vi "Kinect_to_pixels.vi"(0 "previous_X_pixels":dbl, 1 "current_X_kinect":dbl, 2 "previous_X_kinect":dbl, 3 "previous_Y_pixels":dbl, 4 "current_Y_kinect":dbl, 5 "previous_Y_kinect":dbl, 7 "X_Y_speed":dbl, 9 "min_diff":dbl) -> (14 "X_pixels":dbl, 15 "Y_pixels":dbl, 17 "Xmax":dbl=2.5, 18 "Ymax":dbl)   [LabVIEW 2011]
panel:
  out "X_resolution":i16
  out "Y_resolution":i16
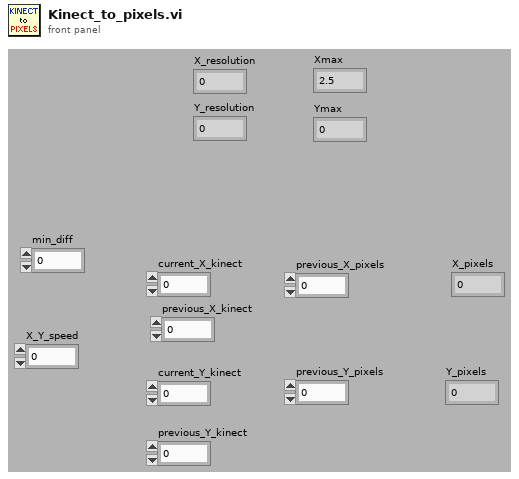
[diagram p1: front panel]
types:
  T1 = typedef "LVAllMonitorsDisplayTypeDef.ctl" = cluster{"Bounds":cluster{"Left":i16, "Top":i16, "Right":i16, "Bottom":i16}, "Depth":i16}[]
  T2 = cluster{"Bounds":cluster{"Left":i16, "Top":i16, "Right":i16, "Bottom":i16}, "Depth":i16}
  T3 = cluster{"Left":i16, "Top":i16, "Right":i16, "Bottom":i16}
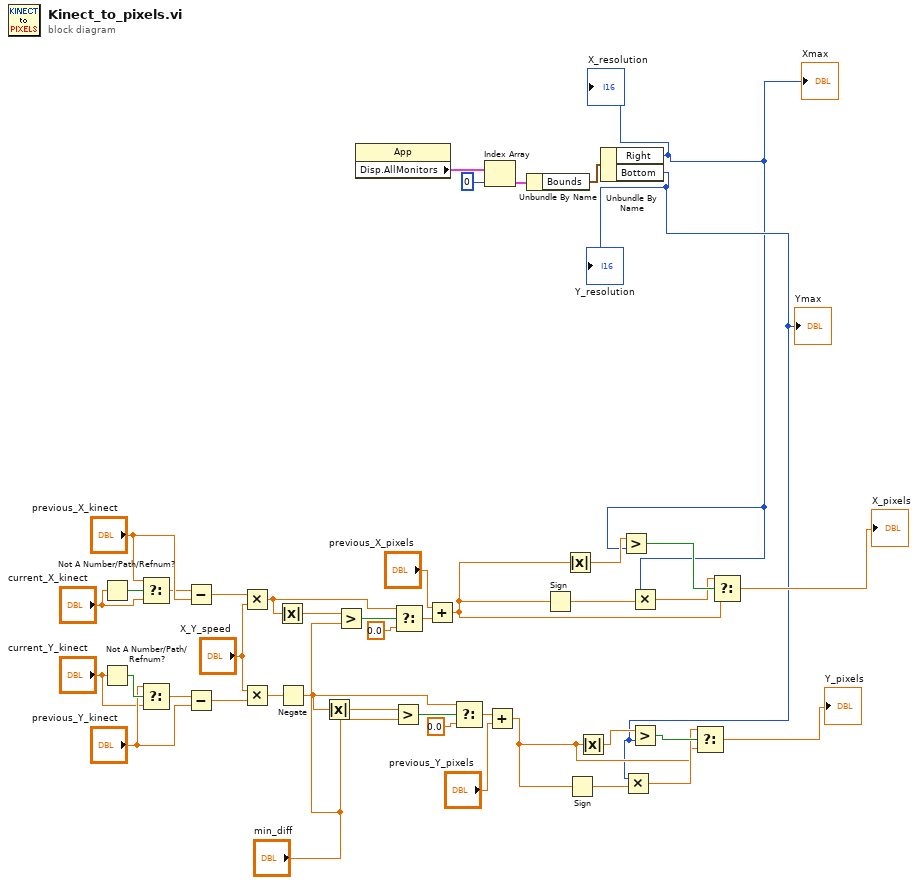
[diagram p0: block diagram]
diagram:
  n1 = Not A Number/Path/Refnum?(number/path/refnum="current_X_kinect") -> (NaN/Path/Refnum?=w22:bool)
  n2 = Not A Number/Path/Refnum?(number/path/refnum="current_Y_kinect") -> (NaN/Path/Refnum?=w18:bool)
  n3 = Select(t="previous_X_kinect", s=w22, f="current_X_kinect") -> (s? t:f=w19:dbl)
  n4 = Select(t="previous_Y_kinect", s=w18, f="current_Y_kinect") -> (s? t:f=w15:dbl)
  n5 = Subtract(x=w19, y="previous_X_kinect") -> (x-y=w39:dbl)
  n6 = Subtract(x=w15, y="previous_Y_kinect") -> (x-y=w38:dbl)
  n7 = Multiply(x=w39, y="X_Y_speed") -> (x*y=w8:dbl)
  n8 = Multiply(x="X_Y_speed", y=w38) -> (x*y=w12:dbl)
  n9 = Absolute Value(x=w8) -> (abs(x)=w7:dbl)
  n10 = Negate(x=w12) -> (-x=w3:dbl)
  n11 = Absolute Value(x=w3) -> (abs(x)=w4:dbl)
  n12 = Greater?(x=w7, y="min_diff") -> (0:w11:bool)
  n13 = property class="App"() -> ("Disp.AllMonitors"=w41:T1)  [unwired: 2 in, 2 out]
  n14 = Greater?(x=w4, y="min_diff") -> (0:w6:bool)
  n15 = Select(t=w8, s=w11, f=0.0) -> (s? t:f=w9:dbl)
  n16 = Add(x="previous_X_pixels", y=w9) -> (x+y=w30:dbl)
  n17 = Select(t=w3, s=w6, f=0.0) -> (s? t:f=w2:dbl)
  n18 = Index Array(array=w41, index=u16 0 ("Front Panel Window:Monitor")) -> (element=w43:T2)
  n19 = Add(x=w2, y="previous_Y_pixels") -> (x+y=w25:dbl)
  n20 = Unbundle By Name(w43) -> ("Bounds"=w40:T3)
  n21 = Sign(1:w30) -> (0:w33:dbl)
  n22 = Absolute Value(x=w30) -> (abs(x)=w35:dbl)
  n23 = Sign(1:w25) -> (0:w27:dbl)
  n24 = Absolute Value(x=w25) -> (abs(x)=w29:dbl)
  n25 = Unbundle By Name(w40) -> ("Right"=w13:i16, "Bottom"=w14:i16)
  "Xmax" <- w13
  "Ymax" <- w14
  "Y_resolution" <- w14
  "X_resolution" <- w13
  n26 = Greater?(x=w35, y=w13) -> (0:w34:bool)
  n27 = Multiply(x=w14, y=w27) -> (x*y=w26:dbl)
  n28 = Multiply(x=w13, y=w33) -> (x*y=w32:dbl)
  n29 = Greater?(x=w29, y=w14) -> (0:w28:bool)
  n30 = Select(t=w26, s=w28, f=w25) -> (s? t:f=→"Y_pixels":dbl)
  n31 = Select(t=w32, s=w34, f=w30) -> (s? t:f=→"X_pixels":dbl)
